vi "Wait Until Act INDI.vi"() -> ()   [LabVIEW 2025]
doc: "Author: Scott Hannahs <sth@magnet.fsu.edu>\n\nThis software is licensed for use under the “MIT License\"\nCopyright (c) 2025 Scott Hannahs, sth@sth@magnet.sthnet.net\n\nPermission is hereby granted, free of charge, to any person obtaining a copy of this software and associated documentation files (the \"Software\"), to deal in the Software without restriction, including without limitation the rights to use, copy, modify, merge, publish, distribute, sublicense, and/or sell copies of the Software, and to permit persons to whom the Software is furnished to do so, subject to the following conditions: The above copyright notice and this permission notice shall be included in all copies or substantial portions of the Software.\n\nTHE SOFTWARE IS PROVIDED \"AS IS\", WITHOUT WARRANTY OF ANY KIND, EXPRESS OR IMPLIED, INCLUDING BUT NOT LIMITED TO THE WARRANTIES OF MERCHANTABILITY, FITNESS FOR A PARTICULAR PURPOSE AND NONINFRINGEMENT. IN NO EVENT SHALL THE AUTHORS OR COPYRIGHT HOLDERS BE LIABLE FOR ANY CLAIM, DAMAGES OR OTHER LIABILITY, WHETHER IN AN ACTION OF CONTRACT, TORT OR OTHERWISE, ARISING FROM, OUT OF OR IN CONNECTION WITH THE SOFTWARE OR THE USE OR OTHER DEALINGS IN THE SOFTWARE."
uses:
  Ctl/Data Acquisition System.ctl
panel:
  in  "Data Acq":T1=enum."NML Data Acquisition-New.vi"
  out "initial value":dbl
  out "monitorng value":dbl
  in  "main":bool
  in  "fire waiting":bool
  in  "update every (s)":dbl=1.0
  in  "Timeout (sec)":dbl=10000.0
  in  "Target Value":dbl
  in  "xxx%":dbl
  in  "index":i32
  in  "Condition":T2(ring)=enum."= target value"
  out "data":dbl[](array[numeric])
  out "error out":errorcluster
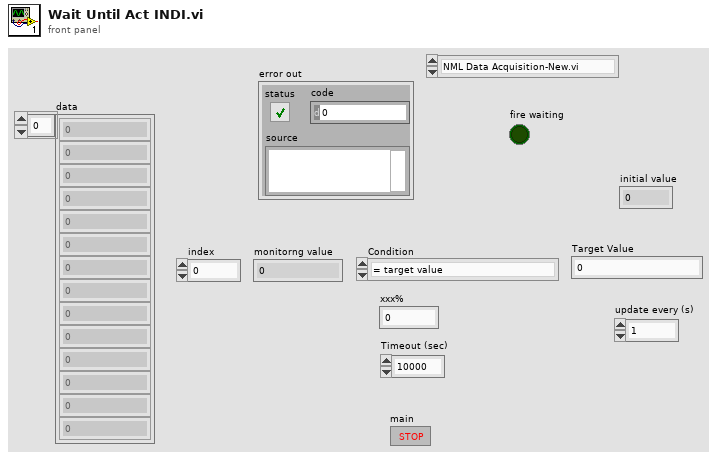
[diagram p1: front panel]
types:
  T1 = typedef "Data Acquisition System.ctl" = enum16{"NML Data Acquisition-old.vi", "NML Data Acquisition-New.vi"}
  T2 = enum16{"within xxx% of target value", "<= target value", ">= target value", "= target value"}
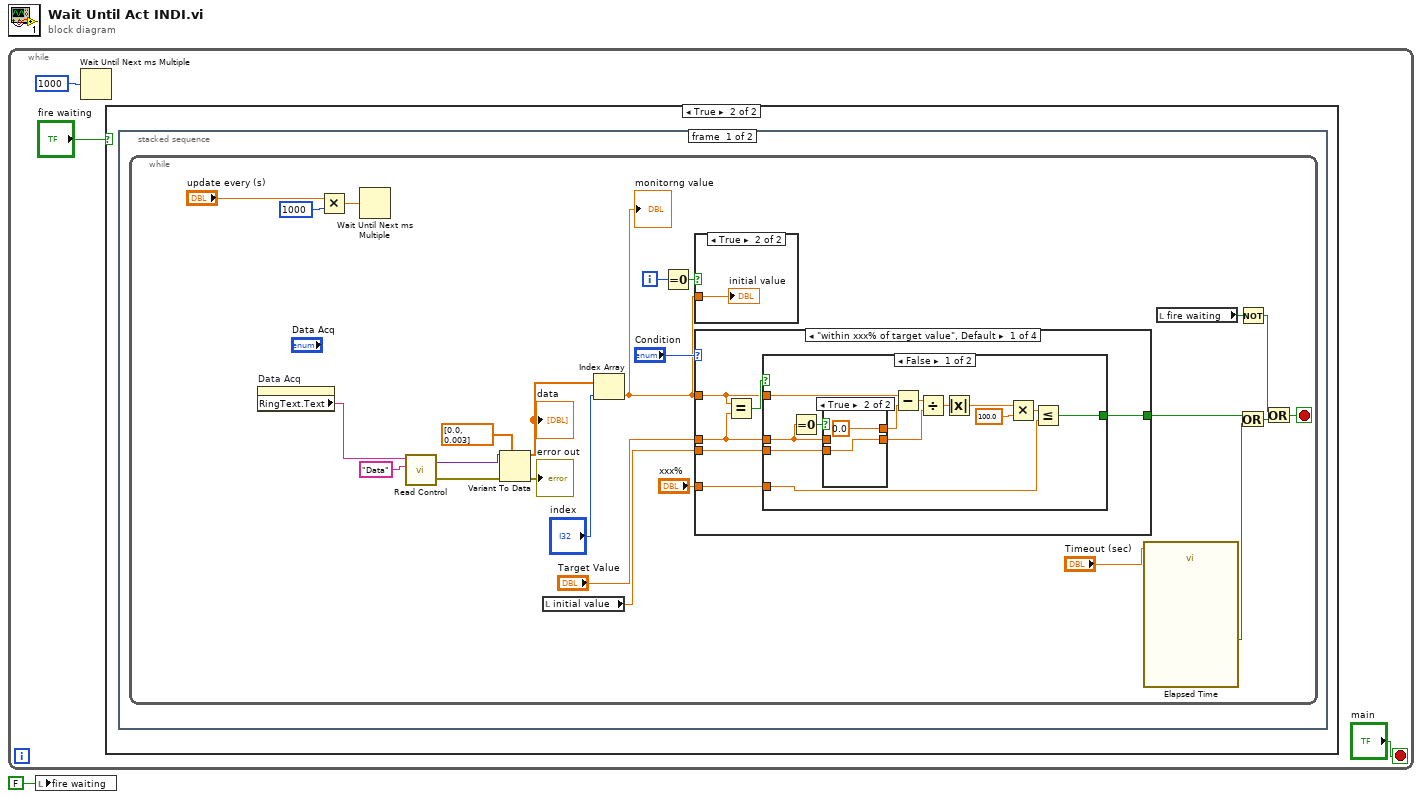
[diagram p0: block diagram]
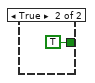
[diagram p5: hidden frame]
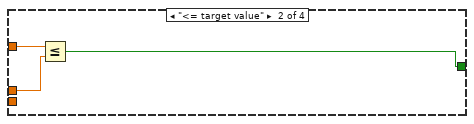
[diagram p6: hidden frame]
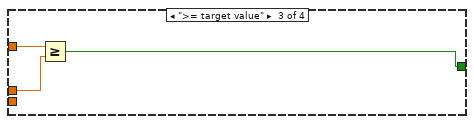
[diagram p7: hidden frame]
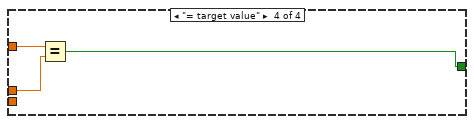
[diagram p8: hidden frame]
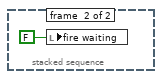
[diagram p9: hidden frame]
diagram:
  n1 = while {
    stop <- "main" stop-if-true
    n2 = Wait Until Next ms Multiple(millisecond multiple=u32 1000) -> ()  [unwired: 1 out]
    n3 = case shown="True" "fire waiting" {
      frame False {
      }
      frame True {
        n4 = stacked-sequence {
          frame #0 {
            n5 = while {
              i -> [w8]
              stop <- w11 stop-if-true
              n6 = property on="Data Acq" class="Enum (strict)"() -> ("RingText.Text"=w5:string)  [unwired: 2 in, 2 out]
              n7 = Multiply(x="update every (s)", y=1000) -> (x*y=w18:dbl)
              n8 = Wait Until Next ms Multiple(millisecond multiple=w18) -> ()  [unwired: 1 out]
              n9 = call "Read Control.vi"("VI Name"=w5, "Control Name"="Data") -> ("Value"=w29:variant, "error out"=w28:errorcluster)  [unwired: 3 in]
              n10 = Variant To Data(error in=w28, type=dbl[] [0.0, 0.003] ("Data"), Variant=w29) -> (data=w25:dbl[], error out=→"error out":errorcluster)
              "data" <- w25
              n11 = local read "initial value"() -> (w6:dbl)
              n12 = Index Array(array=w25, index="index") -> (element=w7:dbl)
              "monitorng value" <- w7
              n13 = Equal To 0?(x=w8) -> (x = 0?=w9:bool)
              n14 = case shown="True" w9 {
                tunnel: w7 -> [_ w30]
                frame False {
                }
                frame True {
                  "initial value" <- w30
                }
              }
              n15 = case shown="\"within xxx% of target value\", Default" "Condition" {
                tunnel: "Target Value" -> [w34 w54 w57 w60]
                tunnel: [w35 w56 w59 w62] -> w16
                tunnel: "xxx%" -> [w33 _ _ _]
                tunnel: w7 -> [w32 w55 w58 w61]
                tunnel: w6 -> [w31 _ _ _]
                frame "within xxx% of target value", Default {
                  n16 = Equal?(x=w32, y=w34) -> (x = y?=w36:bool)
                  n17 = case shown="False" w36 {
                    tunnel: [w41 TRUE] -> w35
                    tunnel: w34 -> [w44 _]
                    tunnel: w33 -> [w45 _]
                    tunnel: w32 -> [w38 _]
                    tunnel: w31 -> [w37 _]
                    frame False {
                      n18 = Equal To 0?(x=w44) -> (x = 0?=w49:bool)
                      n19 = case shown="True" w49 {
                        tunnel: [w50 0.0 ("Target Value")] -> w40
                        tunnel: w44 -> [w50 _]
                        tunnel: [w50 w51] -> w39
                        tunnel: w37 -> [_ w51]
                        frame False {
                        }
                        frame True {
                        }
                      }
                      n20 = Subtract(x=w38, y=w40) -> (x-y=w42:dbl)
                      n21 = Divide(x=w42, y=w39) -> (x/y=w43:dbl)
                      n22 = Absolute Value(x=w43) -> (abs(x)=w46:dbl)
                      n23 = Multiply(x=w46, y=100.0) -> (x*y=w47:dbl)
                      n24 = Less Or Equal?(x=w47, y=w45) -> (x <= y?=w41:bool)
                    }
                    frame True {
                    }
                  }
                }
                frame "<= target value" {
                  n25 = Less Or Equal?(x=w55, y=w54) -> (x <= y?=w56:bool)
                }
                frame ">= target value" {
                  n26 = Greater Or Equal?(x=w58, y=w57) -> (x >= y?=w59:bool)
                }
                frame "= target value" {
                  n27 = Equal?(x=w61, y=w60) -> (x = y?=w62:bool)
                }
              }
              n28 = call "Elapsed Time"("Time Target (s)"="Timeout (sec)") -> ("Time has Elapsed"=w15:bool)  [unwired: 11 in, 7 out]
              n29 = local read "fire waiting"() -> (w14:bool)
              n30 = Not(x=w14) -> (.not. x?=w12:bool)
              n31 = Or(x=w16, y=w15) -> (x .or. y?=w13:bool)
              n32 = Or(x=w12, y=w13) -> (x .or. y?=w11:bool)
            }
          }
          frame #1 {
            n33 = local write "fire waiting"(FALSE ("waiting")) -> ()
          }
        }
      }
    }
  }
  n34 = local write "fire waiting"(FALSE ("fire waiting")) -> ()
